vi "Part 2.vi"() -> ()   [LabVIEW 2016]
panel:
  in  "stop":bool
  in  "S4":bool
  in  "S3":bool
  in  "S2":bool
  in  "S1":bool
  out "LED 2":bool
  out "LED 1":bool
  # "FRONT"
  # "REAR"
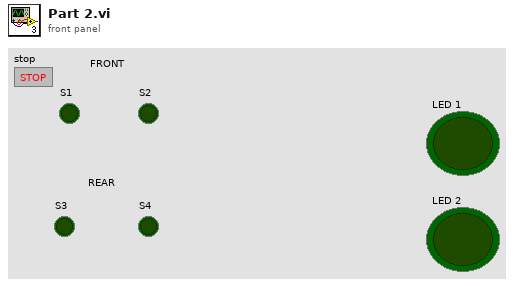
[diagram p1: front panel]
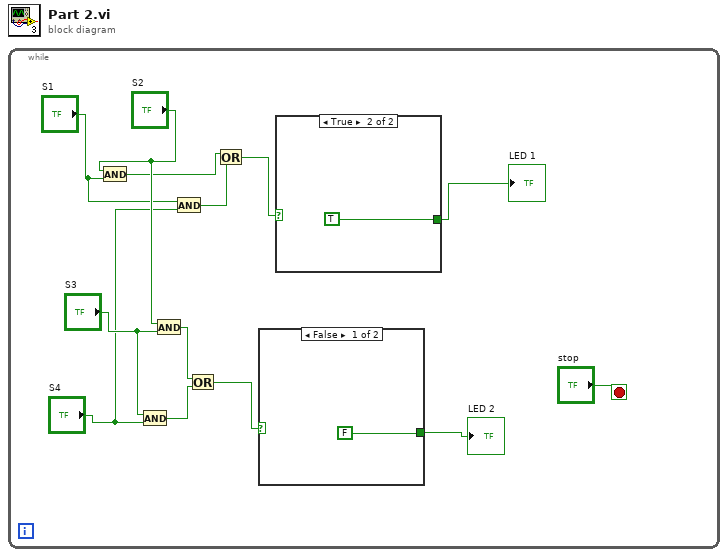
[diagram p0: block diagram]
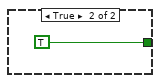
[diagram p2: hidden frame]
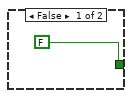
[diagram p3: hidden frame]
diagram:
  n1 = while {
    stop <- "stop" stop-if-true
    n2 = And(x="S2", y="S1") -> (x .and. y?=w5:bool)
    n3 = And(x="S3", y="S4") -> (x .and. y?=w7:bool)
    n4 = And(x="S2", y="S3") -> (x .and. y?=w9:bool)
    n5 = And(x="S1", y="S4") -> (x .and. y?=w4:bool)
    n6 = Or(x=w9, y=w7) -> (x .or. y?=w6:bool)
    n7 = Or(x=w5, y=w4) -> (x .or. y?=w3:bool)
    n8 = case shown="False" w6 {
      tunnel: [FALSE TRUE] -> w11
      frame False {
      }
      frame True {
      }
    }
    "LED 2" <- w11
    n9 = case shown="True" w3 {
      tunnel: [FALSE TRUE] -> w12
      frame False {
      }
      frame True {
      }
    }
    "LED 1" <- w12
  }
